vi "Histogram to CDF.vi"(0 "Histogram":cluster{"Axis":dbl[], "Histogram":dbl[]}, 2 "Normalization Factor":dbl, 3 "Error In":errorcluster) -> (6 "CDF":cluster{"Axis":dbl[], "CDF":dbl[]}, 9 "Error Out":errorcluster)   [LabVIEW 2021, in "Histograms.lvlib"]
doc: "Computes the Cumulative Density Function (<B>CDF</B>) corresponding to the input <B>Histogram</B>.\n\nIf the <B>Normalization Factor</B> is positive, the sum of all histogram bins divided by <B>Normalization Factor</B> is the last value of the CDF.\n\nOtheriwise, the last CDF value is equal to 1."
uses:
  Histograms.lvlib
panel:
  # "see the License on the block diagram (Ctrl+E or Window:Show Block Diagram)"
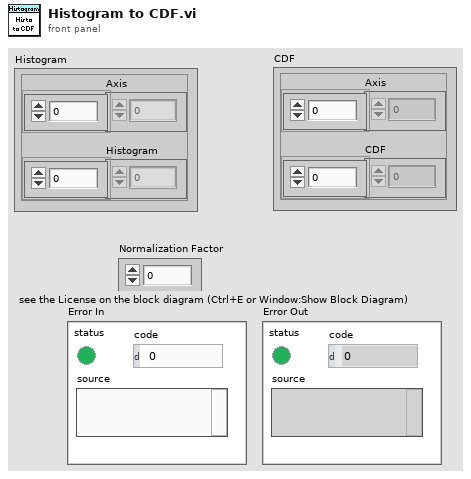
[diagram p1: front panel]
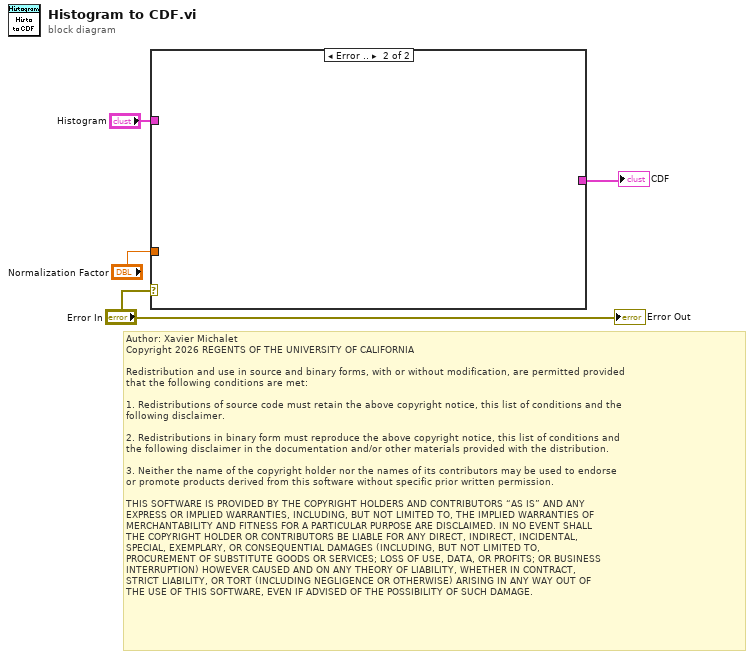
[diagram p0: block diagram]
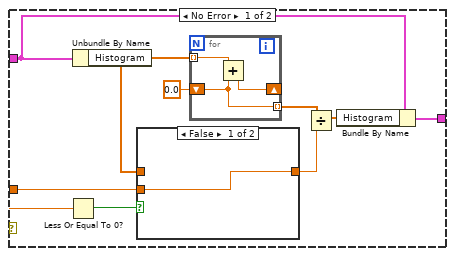
[diagram p2: hidden frame]
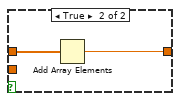
[diagram p3: hidden frame]
diagram:
  # "Author: Xavier Michalet\nCopyright 2026 REGENTS OF THE UNIVERSITY OF CALIFORNIA\n\nRedistribution and use in source and binary forms, with or without modification, are permitted provided\nthat the following conditions are met:\n\n1. Redistributions of source code must retain the above copyright notice, this list of conditions and the\nfollowing disclaimer.\n\n2. Redistributions in binary form must reproduce the above copyright notice, this list of conditions and\nthe following disclaimer in the documentation and/or other materials provided with the distribution.\n\n3. Neither the name of the copyright holder nor the names of its contributors may be used to endorse \nor promote products derived from this software without specific prior written permission.\n\nTHIS SOFTWARE IS PROVIDED BY THE COPYRIGHT HOLDERS AND CONTRIBUTORS “AS IS” AND ANY \nEXPRESS OR IMPLIED WARRANTIES, INCLUDING, BUT NOT LIMITED TO, THE IMPLIED WARRANTIES OF\nMERCHANTABILITY AND FITNESS FOR A PARTICULAR PURPOSE ARE DISCLAIMED. IN NO EVENT SHALL\nTHE COPYRIGHT HOLDER OR CONTRIBUTORS BE LIABLE FOR ANY DIRECT, INDIRECT, INCIDENTAL, \nSPECIAL, EXEMPLARY, OR CONSEQUENTIAL DAMAGES (INCLUDING, BUT NOT LIMITED TO, \nPROCUREMENT OF SUBSTITUTE GOODS OR SERVICES; LOSS OF USE, DATA, OR PROFITS; OR BUSINESS\nINTERRUPTION) HOWEVER CAUSED AND ON ANY THEORY OF LIABILITY, WHETHER IN CONTRACT, \nSTRICT LIABILITY, OR TORT (INCLUDING NEGLIGENCE OR OTHERWISE) ARISING IN ANY WAY OUT OF\nTHE USE OF THIS SOFTWARE, EVEN IF ADVISED OF THE POSSIBILITY OF SUCH DAMAGE."
  n1 = case shown="Error .." "Error In" {
    tunnel: "Histogram" -> [w8 _]
    tunnel: [w7 _] -> w3
    tunnel: "Normalization Factor" -> [w5 _]
    frame No Error {
      n2 = Less Or Equal To 0?(x=w5) -> (x <= 0?=w6:bool)
      n3 = Unbundle By Name(w8) -> ("Histogram"=w12:dbl[])
      n4 = case shown="False" w6 {
        tunnel: w12 -> [_ w16]
        tunnel: [w14 w15] -> w10
        tunnel: w5 -> [w14 _]
        frame False {
        }
        frame True {
          n5 = Add Array Elements(numeric array=w16) -> (sum=w15:dbl)
        }
      }
      n6 = for {
        tunnel: w12 -> [w19] mode=indexing
        shift-right: [w18] -> _
        shift-left: 0.0 -> [w17]
        tunnel: [w17] -> w11 mode=indexing
        n7 = Add(x=w19, y=w17) -> (x+y=w18:dbl)
      }
      n8 = Divide(x=w11, y=w10) -> (x/y=w9:dbl[])
      n9 = Bundle By Name(cluster=w8, "Histogram"=w9) -> (w7:cluster{"Axis":dbl[], "Histogram":dbl[]})
    }
    frame Error {
    }
  }
  "CDF" <- w3
  "Error Out" <- "Error In"
